vi "CRYLogin setup.vi"(6 "Confirm":string caption="aaa", 7 "New PW":bool, 8 "Ask":bool, 9 "New password":string caption="aaa") -> (0 "Cancelled?":bool=TRUE, 1 "New PW?":bool, 2 "Remember?":bool, 3 "Password":string)   [LabVIEW 2013]
panel:
  in  "Cancel":bool
  in  "OK":bool
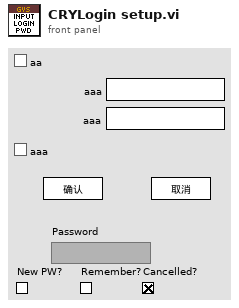
[diagram p1: front panel]
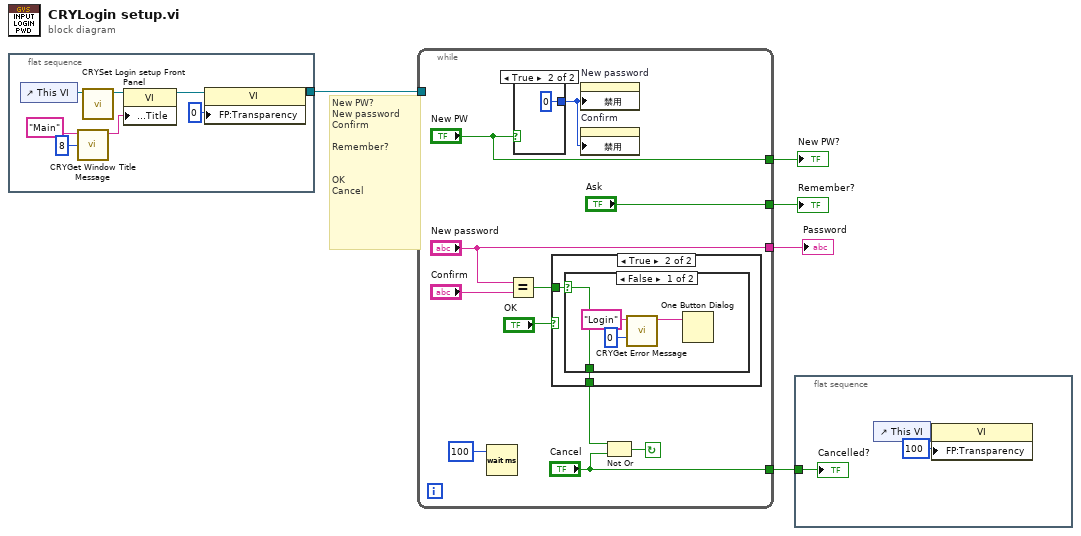
[diagram p0: block diagram]
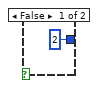
[diagram p2: hidden frame]
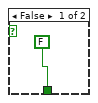
[diagram p3: hidden frame]
diagram:
  # "New PW?\nNew password\nConfirm\n\nRemember?\n\n\nOK\nCancel"
  n1 = flat-sequence {
    tunnel: [w10] -> w1
    frame #0 {
      n2 = control-ref of="This VI"() -> (w13:refnum<vi>)
      n3 = call "CRYGet Window Title Message.vi"("No"=8, "Kind"="Main") -> ("Multibyte String"=w6:string)  [unwired: 4 in, 5 out]
      n4 = call "CRYSet Login setup Front Panel.vi"("Vi Ref in"=w13) -> ("Vi Ref out"=w11:refnum<vi>)  [unwired: 10 in]
      n5 = property class="VI"(reference=w11, "Front Panel.Title"=w6) -> (reference out=w9:refnum<vi>)  [unwired: 1 in, 1 out]
      n6 = property class="VI"(reference=w9, "FP:Transparency"=u8 0 ("Front Panel Window:Transparency")) -> (reference out=w10:refnum<vi>)  [unwired: 1 in, 1 out]
    }
  }
  n7 = while {
    tunnel: ["Cancel"] -> w4
    tunnel: ["New password"] -> w3
    tunnel: ["Ask"] -> w5
    tunnel: ["New PW"] -> w2
    tunnel: w1 -> [_]
    stop <- w23 continue-if-true
    n8 = Wait (ms)(milliseconds to wait=u32 100) -> ()  [unwired: 1 out]
    n9 = Equal?(x="New password", y="Confirm") -> (x = y?=w18:bool)
    n10 = case shown="True" "New PW" {
      tunnel: [u8 2 ("Disabled") u8 0 ("Disabled")] -> w15
      frame False {
      }
      frame True {
      }
    }
    n11 = case shown="True" "OK" {
      tunnel: w18 -> [_ w29]
      tunnel: [FALSE w28] -> w16
      frame False {
      }
      frame True {
        n12 = case shown="False" w29 {
          selector: w29 -> [w33 w34]
          tunnel: [w33 w34] -> w28
          frame False {
            n13 = call "CRYGet Error Message.vi"("Error No"=0, "Kind"="Login") -> ("Message"=w30:string)  [unwired: 4 in, 5 out]
            n14 = One Button Dialog(message=w30) -> ()  [unwired: 2 out]
          }
          frame True {
          }
        }
      }
    }
    n15 = property on="New password" class="Str"("禁用"=w15) -> ()  [unwired: 2 in, 2 out]
    n16 = property on="Confirm" class="Str"("禁用"=w15) -> ()  [unwired: 2 in, 2 out]
    n17 = Not Or(1:"Cancel", 2:w16) -> (0:w23:bool)
  }
  "Password" <- w3
  "Remember?" <- w5
  "New PW?" <- w2
  n18 = flat-sequence {
    tunnel: w4 -> [w37]
    frame #0 {
      n19 = control-ref of="This VI"() -> (w36:refnum<vi>)
      n20 = property class="VI"(reference=w36, "FP:Transparency"=u8 100 ("Front Panel Window:Transparency")) -> ()  [unwired: 1 in, 2 out]
      "Cancelled?" <- w37
    }
  }
